vi "SVT Idle Channel Noise (Frequency) (1 Ch).vi"(0 "complex spectrum":T7={"complex spectrum response"={"f0"=0.0, "df"=1.0, "complex spectrum"=[]}, "spectrum info"={"channel name"="", "description"="", "x-axis units"=0, "spectral info"={"spectrum type"=enum."Power [Magnitude^2]", "linear/dB"=enum."linear", "window"=0, "window size"=0, "FFT size"=0}, "engineering units"=0, "custom label"="", "dB reference [EU]"=0.0, "peak units"=enum."rms", "weighting filter"=0, "spectral density?"=FALSE, "unit label"="", "spectrum skewed?"=FALSE, "complimentary spectrum units"=enum."none"}} {"spectrum info"."x-axis units" items=["Time (s)"=0, "Frequency-CB (Hz)"=1, "Frequency-CPB (Hz)"=1248, "Frequency-Arbitrary (Hz)"=2357, "Quefrency (s)"=2, "Revolutions (rev)"=3, "Order"=4, "Speed (RPM)"=11, "Speed (rad/s)"=21, "Index"=65535]; "spectrum info"."weighting filter" items=["Linear", "A-weighting", "B-weighting", "C-weighting", "ITU-R 468-4", "Dolby", "CCITT", "C-message", "Wb", "Wc", "Wd", "We", "Wf", "Wh", "Wj", "Wk", "Wm", "AES17 20 kHz lowpass", "AES17 40 kHz lowpass", "AES17 20 kHz highpass", "AES17 40 kHz highpass"]; "spectrum info"."dB reference [EU]" format="%.2f"; "spectrum info"."engineering units" items=["custom..."=0, "V"=1, "A"=21, "C"=30, "pC"=31, "s"=32, "-"=29, "Pa"=2, "N"=20, "g"=3, "m/s^2"=4, "m/s"=5, "m"=6, "mm/s"=12, "mm"=13, "micron/s"=14, "micron"=15, "in/s^2"=7, "in/s"=8, "in"=9, "mil/s"=10, "mil"=11, "rad/s^2"=16, "rad/s"=17, "rad"=18, "deg/s^2"=26, "deg/s"=27, "deg"=28, "RPM"=22, "cycle/s^2"=23, "Hz"=24, "cycle"=25, "strain"=19]; "spectrum info"."spectral info"."window" items=["None "=0, "Hanning"=1, "Hamming"=2, "Blackman-Harris"=3, "Exact Blackman"=4, "Blackman"=5, "Flat Top"=6, "4 Term B-Harris "=7, "7 Term B-Harris"=8, "Low Sidelobe"=9, "Force - Exponential"=10, "Gaussian"=62]; "complex spectrum response"."complex spectrum" format="%.2f"; "complex spectrum response"."df" format="%.2f"; "complex spectrum response"."f0" format="%.2f"}, 2 "frequency range":T9={"start frequency"=-1.0, "stop frequency"=-1.0} {"stop frequency" format="%.2f"; "start frequency" format="%.2f"}, 4 "full-scale level [EU rms]":dbl=nan format="%.2f", 5 "error in (no error)":errorcluster, 6 "desired units":T8) -> (11 "average noise level [EU / sqrt(Hz)]":dbl=nan format="%.2f", 12 "unit labels":cluster{"idle channel noise unit label":string}, 13 "maximum spur [EU rms]":cluster{"frequency":dbl, "value":dbl} {"value" format="%.2f"; "frequency" format="%.2f"}, 14 "complex spectrum":T7={"complex spectrum response"={"f0"=0.0, "df"=1.0, "complex spectrum"=[]}, "spectrum info"={"channel name"="", "description"="", "x-axis units"=0, "spectral info"={"spectrum type"=enum."Power [Magnitude^2]", "linear/dB"=enum."linear", "window"=0, "window size"=0, "FFT size"=0}, "engineering units"=0, "custom label"="", "dB reference [EU]"=0.0, "peak units"=enum."rms", "weighting filter"=0, "spectral density?"=FALSE, "unit label"="", "spectrum skewed?"=FALSE, "complimentary spectrum units"=enum."none"}} {"spectrum info"."x-axis units" items=["Time (s)"=0, "Frequency-CB (Hz)"=1, "Frequency-CPB (Hz)"=1248, "Frequency-Arbitrary (Hz)"=2357, "Quefrency (s)"=2, "Revolutions (rev)"=3, "Order"=4, "Speed (RPM)"=11, "Speed (rad/s)"=21, "Index"=65535]; "spectrum info"."weighting filter" items=["Linear", "A-weighting", "B-weighting", "C-weighting", "ITU-R 468-4", "Dolby", "CCITT", "C-message", "Wb", "Wc", "Wd", "We", "Wf", "Wh", "Wj", "Wk", "Wm", "AES17 20 kHz lowpass", "AES17 40 kHz lowpass", "AES17 20 kHz highpass", "AES17 40 kHz highpass"]; "spectrum info"."dB reference [EU]" format="%.2f"; "spectrum info"."engineering units" items=["custom..."=0, "V"=1, "A"=21, "C"=30, "pC"=31, "s"=32, "-"=29, "Pa"=2, "N"=20, "g"=3, "m/s^2"=4, "m/s"=5, "m"=6, "mm/s"=12, "mm"=13, "micron/s"=14, "micron"=15, "in/s^2"=7, "in/s"=8, "in"=9, "mil/s"=10, "mil"=11, "rad/s^2"=16, "rad/s"=17, "rad"=18, "deg/s^2"=26, "deg/s"=27, "deg"=28, "RPM"=22, "cycle/s^2"=23, "Hz"=24, "cycle"=25, "strain"=19]; "spectrum info"."spectral info"."window" items=["None "=0, "Hanning"=1, "Hamming"=2, "Blackman-Harris"=3, "Exact Blackman"=4, "Blackman"=5, "Flat Top"=6, "4 Term B-Harris "=7, "7 Term B-Harris"=8, "Low Sidelobe"=9, "Force - Exponential"=10, "Gaussian"=62]; "complex spectrum response"."complex spectrum" format="%.2f"; "complex spectrum response"."df" format="%.2f"; "complex spectrum response"."f0" format="%.2f"}, 16 "idle channel noise":dbl=nan format="%.2f", 17 "median noise level [EU / sqrt(Hz)]":dbl=nan format="%.2f", 18 "SNR [dB]":dbl=nan format="%.2f", 19 "error out":errorcluster)   [LabVIEW 2017, in "SoundVib_SingleTone.lvlib"]
doc: "Computes idle channel noise, median noise level, and maximum spur of <B>scaled signal</B> and <B>frequency range</B>. This VI also computes the signal-to-noise ratio (SNR) measured without a signal, provided you supply a <B>full-scale level</B>. Wire data to the <B>scaled signal [EU]</B> input to determine the polymorphic instance to use or manually select the instance."
uses:
  <vilib>/addons/Sound and Vibration/svt_Single Tone Measurements/SoundVib_SingleTone.lvlib
  <vilib>/addons/_NISVFA/_Shared subVIs/Controls/svc_Spectrum Info.ctl
  <vilib>/addons/_NISVFA/_Shared subVIs/Controls/svc_X-Axis Units.ctl
  <vilib>/addons/_NISVFA/_Shared subVIs/Controls/svc_Spectrum Type.ctl
  <vilib>/addons/_NISVFA/_Shared subVIs/Controls/svc_Engineering Units Text Ring.ctl
  <vilib>/addons/_NISVFA/_Shared subVIs/Controls/svc_Weighting Filter Text Ring.ctl
  <vilib>/addons/_NISVFA/_Shared subVIs/Controls/svc_Complimentary Spectrum Units.ctl
  <vilib>/addons/_NISVFA/_Spectrum Processing/SVFA Get Spectrum Subset (1 Ch).vi
  <vilib>/addons/_NISVFA/_Spectrum Processing/SVFA Power in Band (1 Ch).vi
  <vilib>/Analysis/baseanly.llb/Mean (DBL).vi
  <vilib>/addons/_NISVFA/_Spectrum Processing/SVFA Unit Conversion (1 Ch).vi
  <vilib>/addons/_NISVFA/_Spectrum Processing/subVIs/svfa_Conversion Utility (spectrum info).vi
  <vilib>/addons/_NISVFA/_Spectrum Processing/subVIs/svfa_Peak to RMS to Peak2Peak.vi
  <vilib>/addons/_NISVFA/_Spectrum Processing/subVIs/svfa_Mag to Mag2.vi
  <vilib>/addons/_NISVFA/_Spectrum Processing/subVIs/svfa_Linear to dB.vi
  <vilib>/addons/_NISVFA/_Spectrum Processing/subVIs/svfa_dBrefA to dBrefB.vi
  <vilib>/addons/_NISVFA/_Spectrum Processing/subVIs/svfa_Spectrum to Spectral Density.vi
  <vilib>/addons/_NISVFA/_Shared subVIs/Common/svc_Get Weighting Enum and Labels.vi
  <vilib>/addons/_NISVFA/_Shared subVIs/Common/svc_Unit Label Lexical Class.vi
  <vilib>/addons/_NISVFA/_Shared subVIs/Common/svc_Engineering Units to Unit Label.vi
  <vilib>/addons/_NISVFA/_Shared subVIs/Common/svc_Format Value (DBL).vi
  <vilib>/addons/_NISVFA/_Spectrum Processing/subVIs/svfa_Spectrum Info Window to windowTd Type Def.vi
  <vilib>/addons/_NISVFA/_Shared subVIs/Common/svc_Build Unit Label for Frequency Range.vi
  <vilib>/addons/_NISVFA/_Shared subVIs/Common/svc_Convert Frequency to Frequency String.vi
  <vilib>/addons/_NISVFA/_Shared subVIs/Common/svc_Check Frequency Range in Spectrum.vi
  <vilib>/addons/_NISVFA/_Spectrum Processing/SVFA Unit Conversion (Complex) (1 Ch).vi
  <vilib>/addons/Sound and Vibration/svt_Distortion/SoundVib_Distortion.lvlib
  <vilib>/Analysis/NI_AALBase.lvlib
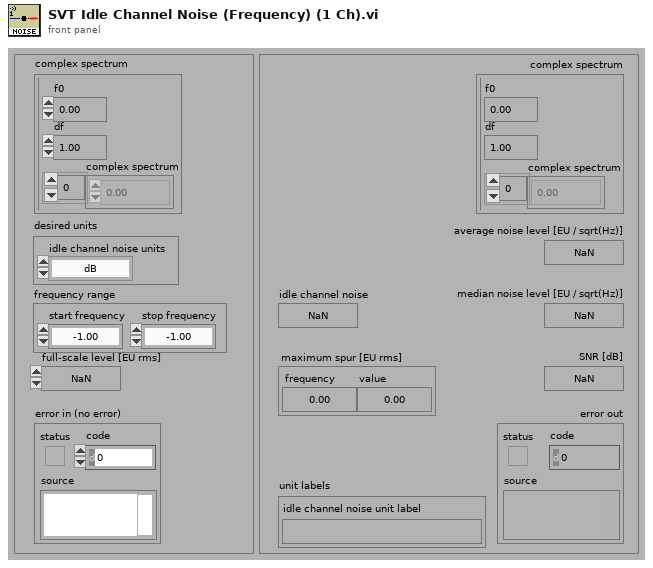
[diagram p1: front panel]
types:
  T1 = typedef "svc_Spectrum Info.ctl" = cluster{"channel name":string, "description":string, "x-axis units":T2, "spectral info":cluster{"spectrum type":T3, "linear/dB":enum16{"linear", "dB"}, "window":u16, "window size":i32, "FFT size":i32}, "engineering units":T4, "custom label":string, "dB reference [EU]":dbl, "peak units":enum16{"rms", "peak", "peak-peak"}, "weighting filter":T5, "spectral density?":bool, "unit label":string, "spectrum skewed?":bool, "complimentary spectrum units":T6}
  T2 = typedef "svc_X-Axis Units.ctl" = u16
  T3 = typedef "svc_Spectrum Type.ctl" = enum16{"FFT Spectrum [complex]", "Amplitude [Magnitude]", "Power [Magnitude^2]", "Cross Spectrum [complex]", "Frequency Response [Complex]"}
  T4 = typedef "svc_Engineering Units Text Ring.ctl" = u16
  T5 = typedef "svc_Weighting Filter Text Ring.ctl" = u16
  T6 = typedef "svc_Complimentary Spectrum Units.ctl" = enum16{"none", "radians", "degrees", "cycles", "imaginary"}
  T7 = cluster{"complex spectrum response":cluster{"f0":dbl, "df":dbl, "complex spectrum":cdb[]}, "spectrum info":T1}
  T8 = cluster{"idle channel noise units":enum16{"dB", "EU^2 rms"}}
  T9 = cluster{"start frequency":dbl, "stop frequency":dbl}
  T10 = cluster{"linear/dB":enum16{"no change", "linear", "dB"}, "dB reference (0: no change)":dbl, "power/magnitude":enum16{"no change", "power", "magnitude"}, "view":enum16{"no change", "rms", "peak", "peak-peak"}}
  T11 = cluster{"power in band":dbl, "power in band":dbl}
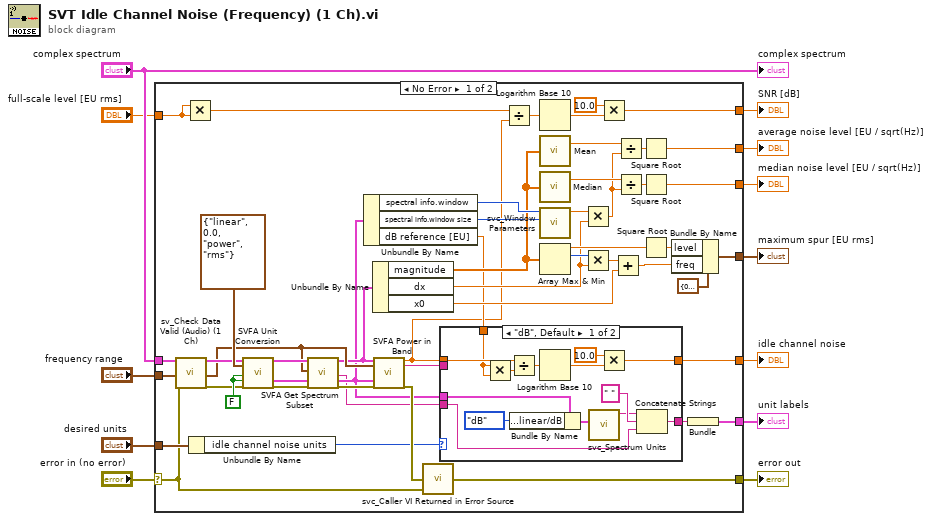
[diagram p0: block diagram]
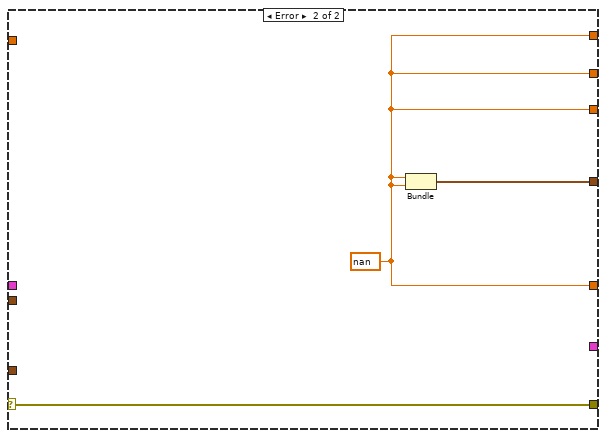
[diagram p3: hidden frame]
diagram:
  n1 = case shown="No Error" "error in (no error)" {
    selector: "error in (no error)" -> [w31 w82]
    tunnel: "complex spectrum" -> [w60 _]
    tunnel: [w61 w82] -> w12
    tunnel: [w17 w80] -> w11
    tunnel: "frequency range" -> [w59 _]
    tunnel: "desired units" -> [w63 _]
    tunnel: [w62 _] -> w6
    tunnel: "full-scale level [EU rms]" -> [w35 _]
    tunnel: [w20 w80] -> w5
    tunnel: [w33 w80] -> w4
    tunnel: [w32 w81] -> w3
    tunnel: [w23 w80] -> w1
    frame No Error {
      w53 = FALSE ("unwrap phase (F)")
      n2 = call <vilib>:"sv_Check Data Valid (Audio) (1 Ch).vi"("complex spectrum"=w60, "frequency range in"=w59, "error in (no error)"=w31) -> ("complex spectrum"=w51:T7, "frequency range out"=w49:T9, "error out"=w52:errorcluster)  [unwired: 9 in, 5 out]
      n3 = Multiply(x=w35, y=w35) -> (x*y=w47:dbl)
      n4 = Unbundle By Name(w63) -> ("idle channel noise units"=w48:enum16{"dB", "EU^2 rms"})
      n5 = call-poly <vilib>:"SVFA Unit Conversion.vi"("complex spectrum"=w51, "desired scaling"=T10 {"linear/dB"=enum."linear", "dB reference (0: no change)"=0.0, "power/magnitude"=enum."power", "view"=enum."rms"}, "unwrap phase (F)"=w53, "convert to degree (T)"=w53, "error in (no error)"=w52) -> ("converted spectrum"=w54:cluster{"x0":dbl, "dx":dbl, "magnitude":dbl[]}, "spectrum info out"=w55:T1, "error out"=w56:errorcluster)  [unwired: 9 in, 3 out]
      n6 = call-poly <vilib>:"SVFA Get Spectrum Subset.vi"("spectrum"=w54, "range"=w49, "spectrum info"=w55, "error in (no error)"=w56) -> ("spectrum subset"=w36:cluster{"x0":dbl, "dx":dbl, "magnitude":dbl[]}, "range label"=w14:string, "dup spectrum info"=w34:T1, "error out"=w50:errorcluster)  [unwired: 10 in, 2 out]
      n7 = Unbundle By Name(w34) -> ("spectral info.window"=w41:u16, "spectral info.window size"=w19:i32, "dB reference [EU]"=w18:dbl)
      n8 = Unbundle By Name(w36) -> ("magnitude"=w30:dbl[], "dx"=w26:dbl, "x0"=w44:dbl)
      n9 = call-poly <vilib>:"SVFA Power in Band.vi"("spectrum"=w36, "range"=w49, "spectrum info"=w34, "error in (no error)"=w50) -> ("power in band"=w13:dbl, "unit label"=w15:string, "error out"=w58:errorcluster)  [unwired: 13 in]
      n10 = call <vilib>:"svc_Caller VI Returned in Error Source.vi"("warning input to caller"=w31, "error in (no error)"=w58) -> ("error out"=w61:errorcluster)  [unwired: 3 in]
      n11 = case shown="\"dB\", Default" w48 {
        tunnel: w34 -> [w77 _]
        tunnel: w13 -> [w70 w79]
        tunnel: w18 -> [w69 _]
        tunnel: [w68 w79] -> w17
        tunnel: [w64 w78] -> w16
        tunnel: w15 -> [_ w78]
        tunnel: w14 -> [w65 _]
        frame "dB", Default {
          n12 = Multiply(x=w69, y=w69) -> (x*y=w71:dbl)
          n13 = Divide(x=w70, y=w71) -> (x/y=w72:dbl)
          n14 = Bundle By Name(cluster=w77, "spectral info.linear/dB"=enum16{"linear", "dB"}."dB") -> (w76:T1)
          n15 = Logarithm Base 10(1:w72) -> (0:w74:dbl)
          n16 = call <vilib>:"svc_Spectrum Units.vi"("spectrum info in"=w76) -> ("unit label"=w66:string)  [unwired: 3 in, 3 out]
          n17 = Multiply(x=10.0, y=w74) -> (x*y=w68:dbl)
          n18 = Concatenate Strings(w66, " " ("string"), w65) -> (w64:string)
        }
        frame "EU^2 rms" {
        }
      }
      n19 = Divide(x=w47, y=w13) -> (x/y=w38:dbl)
      n20 = Logarithm Base 10(1:w38) -> (0:w22:dbl)
      n21 = call-poly <vilib>:"Mean.vi"("X"=w30) -> ("mean"=w28:dbl)  [unwired: 1 out]
      n22 = call <vilib>:"Median.vi"("X"=w30) -> ("median"=w40:dbl)  [unwired: 1 out]
      n23 = call <vilib>:"svc_Window Parameters.vi"("window size"=w19, "window"=w41) -> ("ENBW"=w42:dbl)  [unwired: 6 in, 3 out]
      n24 = Array Max & Min(array=w30) -> (max value=w43:dbl, max index (indices)=w46:i32)  [unwired: 2 out]
      n25 = Multiply(x=w42, y=w26) -> (x*y=w27:dbl)
      n26 = Multiply(x=w46, y=w26) -> (x*y=w45:dbl)
      n27 = Multiply(x=10.0, y=w22) -> (x*y=w20:dbl)
      n28 = Add(x=w45, y=w44) -> (x+y=w24:dbl)
      n29 = Divide(x=w28, y=w27) -> (x/y=w29:dbl)
      n30 = Divide(x=w40, y=w27) -> (x/y=w39:dbl)
      n31 = Square Root(x=w29) -> (sqrt(x)=w23:dbl)
      n32 = Square Root(x=w39) -> (sqrt(x)=w33:dbl)
      n33 = Square Root(x=w43) -> (sqrt(x)=w37:dbl)
      n34 = Bundle By Name(cluster=cluster{"freq":dbl, "level":dbl} {"freq"=0.0, "level"=0.0} ("maximum spur [EU rms]"), "level"=w37, "freq"=w24) -> (w32:cluster{"freq":dbl, "level":dbl})
      n35 = Bundle("unit label"=w16) -> (w62:cluster{"unit label":string})  [unwired: 1 in]
    }
    frame Error {
      w80 = nan ("power in band")
      n36 = Bundle("power in band"=w80, "power in band"=w80) -> (w81:T11)  [unwired: 1 in]
    }
  }
  "error out" <- w12
  "idle channel noise" <- w11
  "unit labels" <- w6
  "maximum spur [EU rms]" <- w3
  "SNR [dB]" <- w5
  "median noise level [EU / sqrt(Hz)]" <- w4
  "average noise level [EU / sqrt(Hz)]" <- w1
  "complex spectrum" <- "complex spectrum"
